vi "Test rotation mount.vi"() -> ()   [LabVIEW 2018]
uses:
  C:/Project/SerialSectionOCT/SerialSectOCT/Labview Software/Thorlabs.MotionControl.Controls.dll
  Thorlabs.MotionControl.Controls.dll
  Hardware Mfg/Thorlabs Translation Stages/Controls/Translation Stage Cluster.ctl
  General/Controls/Translation Stage Types.ctl
  General/Controls/Set Get Controls.ctl
  Hardware Mfg/Thorlabs Translation Stages/Controls/Motion Translation Module Control2.ctl
  Hardware Mfg/Thorlabs Cage Rotation/refnum control.ctl
panel:
  out "Cluster out":T1
  in  "Cluster In":T1={"Position"=0.0, "Is.Enabled?"=FALSE, "Is.Connected?"=FALSE, "Device SN"="55151324", "AccelerationMaximum"=10.0, "VelocityMaximum"=10.0, "Acceleration"=10.0, "Velocity"=10.0, "waitTimeout (ms)"=10000, "Model"=enum."None", "Is.Homed?"=FALSE, "MOVE"=FALSE}
  in  "LTS Reference":refnum<k24>(container)
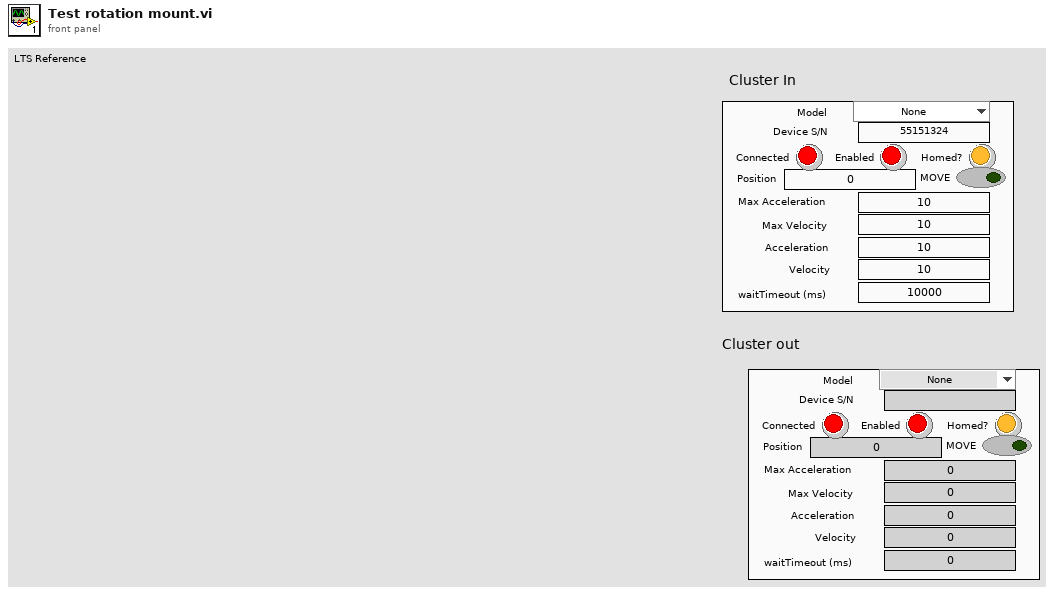
[diagram p1: front panel]
types:
  T1 = typedef "Translation Stage Cluster.ctl" = cluster{"Position":dbl, "Is.Enabled?":bool, "Is.Connected?":bool, "Device SN":string, "AccelerationMaximum":dbl, "VelocityMaximum":dbl, "Acceleration":dbl, "Velocity":dbl, "waitTimeout (ms)":i32, "Model":T2, "Is.Homed?":bool, "MOVE":bool}
  T2 = typedef "Translation Stage Types.ctl" = enum16{"None", "Thorlabs LTS", "Thorlabs MLJ"}
  T3 = typedef "Motion Translation Module Control2.ctl" = enum16{"Init", "Home", "Status", "Velocity/Accel", "Position", "Jog", "Stop", "Uninit", "Enable", "Disable"}
  T4 = typedef "refnum control.ctl" = enum16{"Get", "Init"}
  T5 = typedef "Set Get Controls.ctl" = enum16{"Set", "Get"}
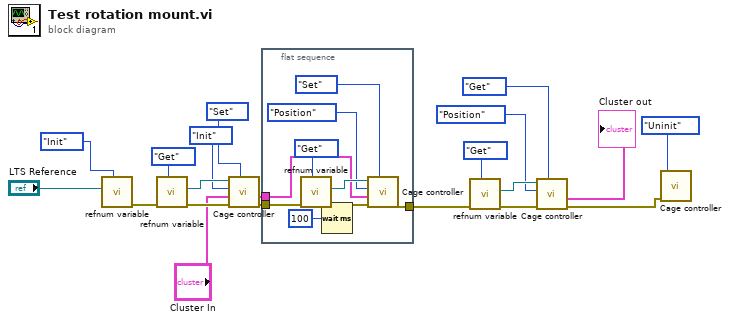
[diagram p0: block diagram]
diagram:
  n1 = call "refnum variable.vi"("action"=refnum_control."Init", "reference in"="LTS Reference") -> ("error out"=w10:errorcluster)  [unwired: 8 in, 1 out]
  n2 = call "refnum variable.vi"("action"=refnum_control."Get", "error in (no error)"=w10) -> ("error out"=w18:errorcluster, "reference in 2"=w17:refnum<k24>)  [unwired: 8 in]
  n3 = call "Cage controller.vi"("Set/Get"=Set_Get_Controls."Set", "error in (no error)"=w18, "Cluster In"="Cluster In", "Action"=Motion_Translation_Module_Control2."Init", "reference in"=w17) -> ("error out"=w14:errorcluster, "Cluster out"=w13:T1)  [unwired: 4 in, 1 out]
  n4 = flat-sequence {
    tunnel: w14 -> [w25]
    tunnel: w13 -> [w24]
    tunnel: [w22] -> w4
    frame #0 {
      n5 = call "refnum variable.vi"("action"=refnum_control."Get", "error in (no error)"=w25) -> ("error out"=w27:errorcluster, "reference in 2"=w26:refnum<k24>)  [unwired: 8 in]
      n6 = Wait (ms)(milliseconds to wait=u32 100) -> ()  [unwired: 1 out]
      n7 = call "Cage controller.vi"("Set/Get"=Set_Get_Controls."Set", "error in (no error)"=w27, "Cluster In"=w24, "Action"=Motion_Translation_Module_Control2."Position", "reference in"=w26) -> ("error out"=w22:errorcluster)  [unwired: 4 in, 2 out]
    }
  }
  n8 = call "refnum variable.vi"("action"=refnum_control."Get", "error in (no error)"=w4) -> ("error out"=w7:errorcluster, "reference in 2"=w6:refnum<k24>)  [unwired: 8 in]
  n9 = call "Cage controller.vi"("Set/Get"=Set_Get_Controls."Get", "error in (no error)"=w7, "Action"=Motion_Translation_Module_Control2."Position", "reference in"=w6) -> ("error out"=w2:errorcluster, "Cluster out"=→"Cluster out":T1)  [unwired: 5 in, 1 out]
  n10 = call "Cage controller.vi"("error in (no error)"=w2, "Action"=Motion_Translation_Module_Control2."Uninit") -> ()  [unwired: 7 in, 3 out]
